vi "p38_vector.vi"() -> ()   [LabVIEW 2013]
uses:
  <vilib>/Analysis/baseanly.llb/Real A x B.vi
  <vilib>/robotics/Kinematics/NI_Kinematics.lvlib
  <vilib>/Analysis/NI_AALBase.lvlib
panel:
  out "Position (X,Y,Z)":dbl[](array[numeric])=[1.0, 1.0, 1.0] format="%#.5f"
  out "rotation matrix":picture
  out "transformation plot":refnum<vi>(3d-picture)
  out "transformation matrix":picture
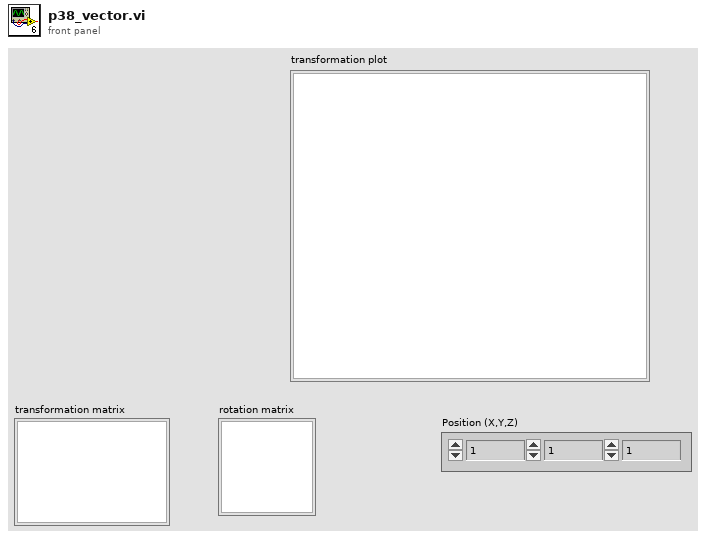
[diagram p1: front panel]
types:
  T1 = typedef "NI_Matrix.lvlib/RealMatrix.ctl" = dbl[][]
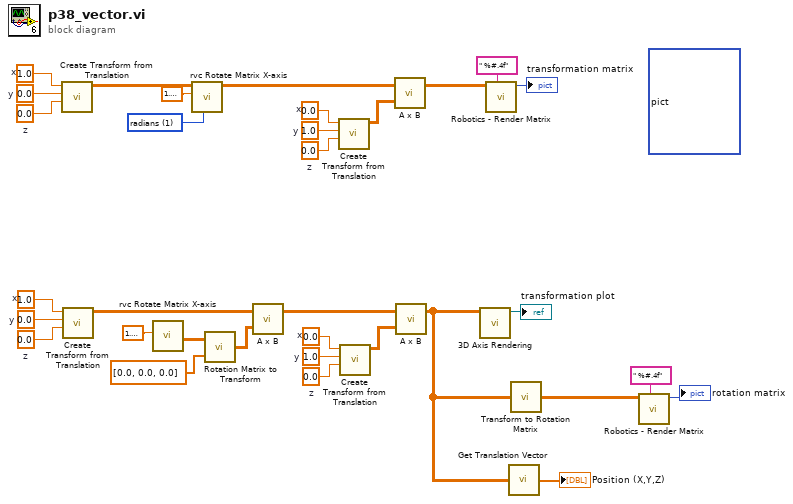
[diagram p0: block diagram]
diagram:
  w1 = u16 1 items=["degree", "radians"] ("angle unit")
  (unwired) picture bytes[806] ("transformation matrix")
  w14 = 0.0  # z
  w15 = 0.0  # x
  w16 = 1.0  # y
  w13 = 0.0  # z
  w12 = 1.0  # x
  w11 = 0.0  # y
  w23 = 0.0  # z
  w22 = 0.0  # x
  w21 = 1.0  # y
  w24 = 0.0  # z
  w25 = 1.0  # x
  w26 = 0.0  # y
  n1 = call <vilib>:"Create Transform from Translation.vi"("z"=w24, "y"=w26, "x"=w25) -> ("transform"=w3:T1)  [unwired: 8 in]
  n2 = call <vilib>:"Create Transform from Translation.vi"("z"=w13, "y"=w11, "x"=w12) -> ("transform"=w6:T1)  [unwired: 8 in]
  n3 = call "rvc Rotate Matrix X-axis.vi"("angle"=1.5707963267948966) -> ("rotation matrix"=w8:T1)  [unwired: 10 in]
  n4 = call "rvc Rotate Matrix X-axis.vi"("angle unit"=w1, "angle"=1.5707963267948966, "rotation matrix in"=w3) -> ("rotation matrix"=w2:T1)  [unwired: 8 in]
  n5 = call <vilib>:"Rotation Matrix to Transform.vi"("translation vector"=dbl[] [0.0, 0.0, 0.0], "rotation matrix"=w8) -> ("transform"=w10:T1)
  n6 = call-poly <vilib>:"A x B.vi"("B"=w10, "A"=w6) -> ("A x B"=w7:T1)  [unwired: 1 out]
  n7 = call <vilib>:"Create Transform from Translation.vi"("z"=w23, "y"=w21, "x"=w22) -> ("transform"=w20:T1)  [unwired: 8 in]
  n8 = call <vilib>:"Create Transform from Translation.vi"("z"=w14, "y"=w16, "x"=w15) -> ("transform"=w17:T1)  [unwired: 8 in]
  n9 = call-poly <vilib>:"A x B.vi"("B"=w20, "A"=w2) -> ("A x B"=w18:T1)  [unwired: 1 out]
  n10 = call-poly <vilib>:"A x B.vi"("B"=w17, "A"=w7) -> ("A x B"=w4:T1)  [unwired: 1 out]
  n11 = call "3D Axis Rendering.vi"("rotation matrix"=w4) -> ("SceneNode out"=→"transformation plot":refnum<vi>)  [unwired: 10 in]
  n12 = call "Robotics - Render Matrix.vi"("format string"=" %#.4f", "A"=w18) -> ("picture out"=→"transformation matrix":picture)  [unwired: 9 in]
  n13 = call <vilib>:"Get Translation Vector.vi"("transform"=w4) -> ("translation vector"=→"Position (X,Y,Z)":dbl[])
  n14 = call <vilib>:"Transform to Rotation Matrix.vi"("transform"=w4) -> ("rotation matrix"=w29:T1)
  n15 = call "Robotics - Render Matrix.vi"("format string"=" %#.4f", "A"=w29) -> ("picture out"=→"rotation matrix":picture)  [unwired: 9 in]
